vi "Adaptive Filter 2.vi"(4 "Beta":fxp<+/-,24,0>, 6 "Noise":T1, 8 "Weights":refnum<k21>="Filter Weights 0", 9 "Taps":refnum<k21>="Filter Taps 0", 11 "Input":fxp<+/-,16,2>) -> (3 "Error Out":fxp<+/-,16,2> format="%.16g")   [LabVIEW 2013]
uses:
  <vilib>/Platform/TimedLoop/XDataNode/timing_clust.ctl
  <vilib>/Platform/TimedLoop/XDataNode/nitl_modes.ctl
  <vilib>/Platform/TimedLoop/XDataNode/wakeup.ctl
  <vilib>/rvi/Emulation/niFpgaSctlEmulationGetInTimedLoop.vi
  <vilib>/rvi/Emulation/niFpgaEmulationReportErrorSimple.vi
  <vilib>/rvi/Emulation/niFpgaGetClockAttributes.vi
  <vilib>/rvi/Emulation/niFpgaCriticalErrorInLSC.vi
  <vilib>/rvi/DataTransferAndStorage/Container/Common/niFpgaContainerExecOnDevCompGetState.vi
  <vilib>/rvi/Memory/Memory_Emulation/nirvimemoryFastEmulationFpgaImpl.vi
  <instcachedir>/0/nirvimemoryFastEmulationFpgaImpl_5FBAB50466BC4C939F684F8805638BFC.lvgen/nirvimemoryFastEmulationFpgaImpl_5FBAB50466BC4C939F684F8805638BFC_002.vi
  <vilib>/rvi/DataTransferAndStorage/Container/Common/niFpgaContainerGetUniqueNameForEmu.vi
  <vilib>/rvi/Memory/Memory_Emulation/niFpgaMemoryEmulationCacheClearOnFirstRun.vi
  <vilib>/rvi/Memory/Memory_Emulation/nirvimemoryEmulationManagerCache_MakeExclusive.vi
  <vilib>/rvi/Memory/Memory_Emulation/niFpgaMemoryEmulationValidateCache.vi
  <vilib>/rvi/Memory/Memory_Emulation/nirvimemoryEmulationManagerCache_ReleaseExclusive.vi
  <vilib>/rvi/Memory/Memory_Emulation/nirvimemoryEmulationManagerCache_InsertValue.vi
  <vilib>/Utility/error.llb/Clear Errors.vi
  <vilib>/rvi/Memory/Memory_Emulation/nirvimemoryEmulationManagerCache_GetValue.vi
  <vilib>/rvi/Memory/Memory_Emulation/nirvimemoryEmulationManagerCache_SetValue.vi
  <vilib>/rvi/Emulation/niFpgaSctlEmulationResourceMgr.vi
  <vilib>/Platform/TimedLoop/XDataNode/XDataNode.xnode
  <vilib>/rvi/DataTransferAndStorage/Container/XNode/niFpgaContainer.xnode
  <vilib>/rvi/Memory/Memory_Emulation/niFpgaMemoryEmulationRefIn.vi
  <vilib>/Platform/TimedLoop/XDataNode/XDNodeRunTimeDep.lvlib
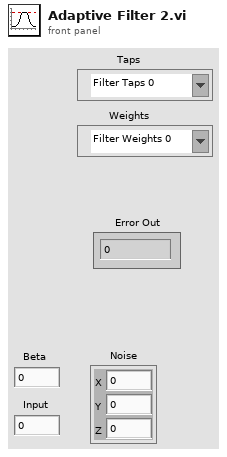
[diagram p1: front panel]
types:
  T1 = cluster{"X":fxp<+/-,16,2>, "Y":fxp<+/-,16,2>, "Z":fxp<+/-,16,2>}
  T2 = typedef "XDNodeRunTimeDep.lvlib/timing_clust.ctl" = cluster{"Expected End [f-1]":u64, "Actual End [f-1]":u64, "Finished Late? [f-1]":bool, "Expected End [i-1]":u64, "Actual End [i-1]":u64, "Finished Late? [i-1]":bool, "Expected Start [i]":u64, "Actual Start [i]":u64, "Expected Start [f]":u64, "Actual Start [f]":u64, "Source Name":string, "Structure Name":string, "Period":i64, "Deadline":i64, "Offset":i64, "Start":i64, "Priority":i32, "Timeout":i32, "Mode":T3, "Wakeup Reason":T4, "Error":errorcluster, "Source Type":string, "Secondary Source Type":string, "Global End Time":u64, "Global Start Time":u64, "Frame Duration":u64, "Iteration Duration":u64, "Assigned CPU":i32, "I/O Scan Engine Mode":u32}
  T3 = typedef "XDNodeRunTimeDep.lvlib/nitl_modes.ctl" = enum32{"No Change", "Process missed periods, maintain original phase", "Discard missed periods, maintain original phase", "Process missed periods, ignore original phase", "Discard missed periods, ignore original phase"}
  T4 = typedef "XDNodeRunTimeDep.lvlib/wakeup.ctl" = enum32{"Normal", "Aborted", "Asynchronous wakeup", "Timing source error", "Timed loop error", "Timeout"}
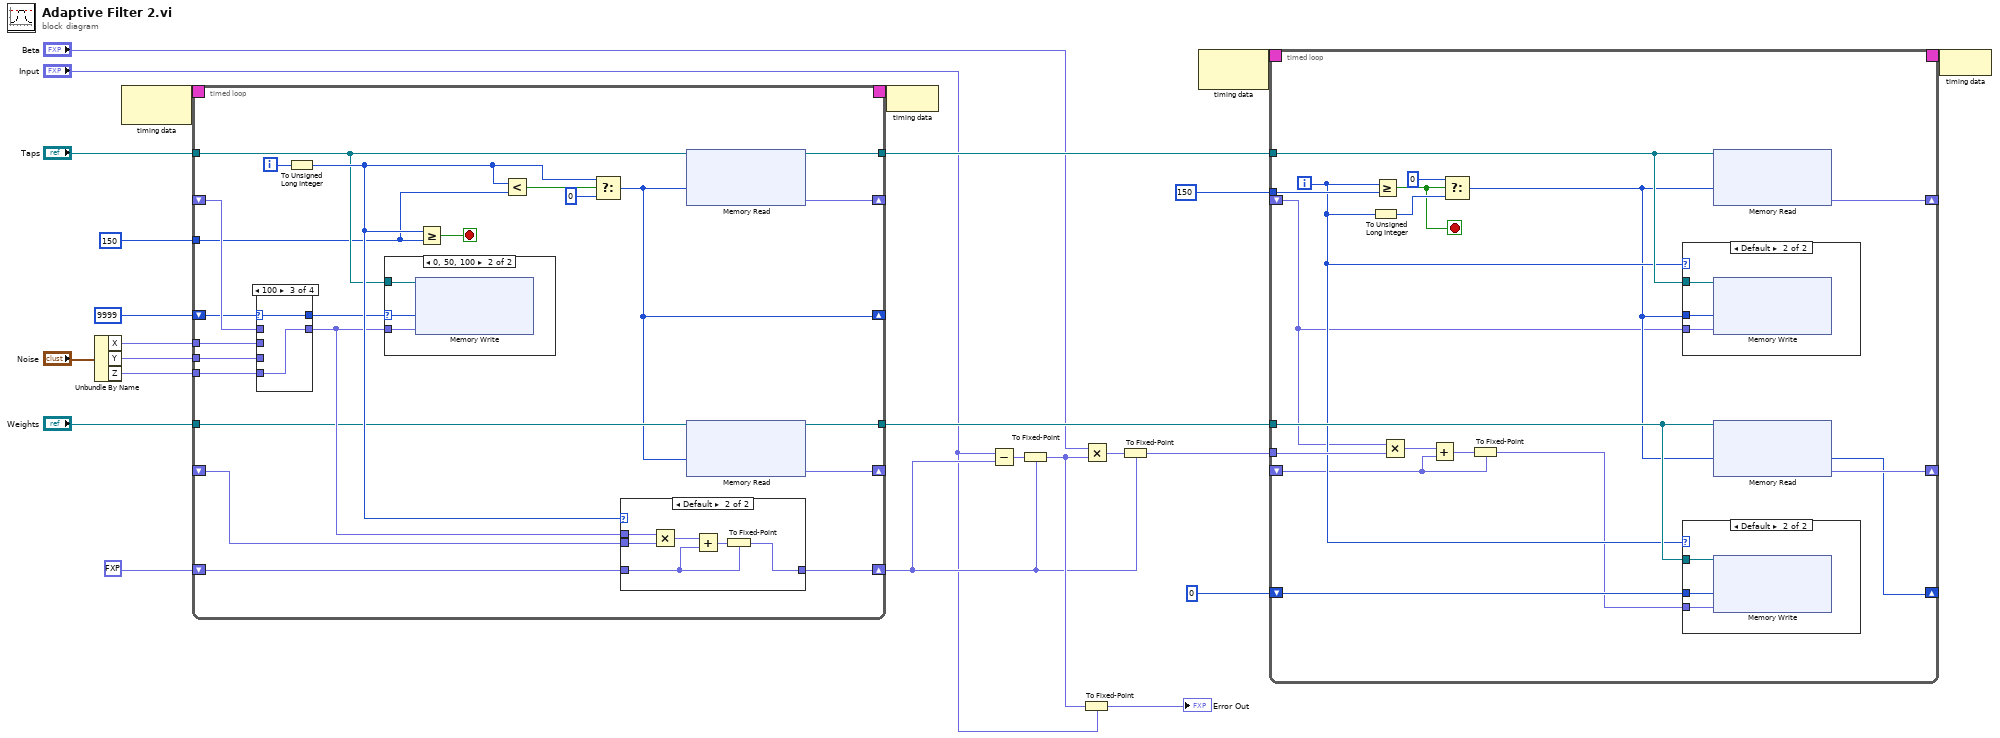
[diagram p0: block diagram]
diagram:
  n1 = Unbundle By Name("Noise") -> ("X"=w24:fxp<+/-,16,2>, "Y"=w23:fxp<+/-,16,2>, "Z"=w22:fxp<+/-,16,2>)
  n2 = node-c288() -> (w15:T2)  [unwired: 1 in]
  n3 = timed-loop {
    tunnel: "Taps" -> [w31]
    tunnel: w24 -> [w48]
    tunnel: w23 -> [w47]
    tunnel: w22 -> [w46]
    tunnel: "Weights" -> [w28]
    shift-right: [w44] -> w2
    shift-left: fxp<+/-,33,5> 0.0 ("x+y") -> [w45]
    tunnel: [w41] -> w11
    tunnel: [w42] -> w18
    timing: w15 -> [_]
    timing-out: [_] -> w14
    shift-right: [w40] -> _
    shift-left: _ -> [w36]
    shift-right: [w27] -> _
    shift-left: _ -> [w39]
    shift-right: [w26] -> _
    shift-left: u32 9999 -> [w35]
    tunnel: u32 150 ("y") -> [w29]
    i -> [w37]
    stop <- w43 stop-if-true
    n4 = case shown="100" w35 {
      selector: w35 -> [w59 w61 w63 w65]
      tunnel: w36 -> [_ _ _ w66]
      tunnel: w48 -> [w60 _ _ _]
      tunnel: w47 -> [_ w62 _ _]
      tunnel: w46 -> [_ _ w64 _]
      tunnel: [w60 w62 w64 w66] -> w30
      tunnel: [w59 w61 w63 w65] -> w32
      frame 0 {
      }
      frame 50 {
      }
      frame 100 {
      }
      frame Default {
      }
    }
    n5 = To Unsigned Long Integer(number=w37) -> (unsigned 32bit integer=w33:u32)
    n6 = case shown="0, 50, 100" w32 {
      selector: w32 -> [_ w49]
      tunnel: w31 -> [_ w51]
      tunnel: w30 -> [_ w50]
      frame Default {
      }
      frame 0, 50, 100 {
        n7 = xnode ("Memory Write")("Address"=w49, "Data"=w50, "Memory In"=w51) -> ()  [unwired: 1 out]
      }
    }
    n8 = Greater Or Equal?(x=w33, y=w29) -> (x >= y?=w43:bool)
    n9 = Less?(x=w33, y=w29) -> (x < y?=w34:bool)
    n10 = Select(t=w33, s=w34, f=u32 0) -> (s? t:f=w26:u32)
    n11 = case shown="Default" w33 {
      tunnel: w45 -> [w52 w56]
      tunnel: [w52 w55] -> w44
      tunnel: w39 -> [_ w54]
      tunnel: w30 -> [_ w53]
      frame 0 {
      }
      frame Default {
        n12 = Multiply(x=w53, y=w54) -> (x*y=w58:fxp<+/-,32,4>)
        n13 = Add(x=w58, y=w56) -> (x+y=w57:fxp<+/-,34,6>)
        n14 = To Fixed-Point(fixed-point type=w56, number=w57) -> (fixed-point=w55:fxp<+/-,33,5>)
      }
    }
    n15 = xnode ("Memory Read")("Address"=w26, "Memory In"=w31) -> ("Data"=w40:fxp<+/-,16,2>, "Memory Out"=w41:refnum<k21>)
    n16 = xnode ("Memory Read")("Address"=w26, "Memory In"=w28) -> ("Data"=w27:fxp<+/-,16,2>, "Memory Out"=w42:refnum<k21>)
  }
  n17 = node-c288(w14) -> ()
  n18 = Subtract(x="Input", y=w2) -> (x-y=w20:fxp<+/-,34,6>)
  n19 = To Fixed-Point(fixed-point type=w2, number=w20) -> (fixed-point=w19:fxp<+/-,33,5>)
  n20 = To Fixed-Point(fixed-point type="Input", number=w19) -> (fixed-point=→"Error Out":fxp<+/-,16,2>)
  n21 = Multiply(x="Beta", y=w19) -> (x*y=w17:fxp<+/-,57,5>)
  n22 = To Fixed-Point(fixed-point type=w2, number=w17) -> (fixed-point=w16:fxp<+/-,33,5>)
  n23 = node-c288() -> (w13:T2)  [unwired: 1 in]
  n24 = timed-loop {
    tunnel: w11 -> [w76]
    tunnel: w18 -> [w80]
    tunnel: w16 -> [w85]
    timing: w13 -> [_]
    timing-out: [_] -> w12
    tunnel: 150 ("y") -> [w83]
    shift-right: [w81] -> _
    shift-left: _ -> [w73]
    shift-right: [w79] -> _
    shift-left: _ -> [w70]
    shift-right: [w74] -> _
    shift-left: u32 0 ("t") -> [w78]
    i -> [w75]
    stop <- w69 stop-if-true
    n25 = To Unsigned Long Integer(number=w75) -> (unsigned 32bit integer=w77:u32)
    n26 = Greater Or Equal?(x=w75, y=w83) -> (x >= y?=w69:bool)
    n27 = Multiply(x=w73, y=w85) -> (x*y=w84:fxp<+/-,49,7>)
    n28 = Add(x=w84, y=w70) -> (x+y=w72:fxp<+/-,49,7>)
    n29 = Select(t=u32 0, s=w69, f=w77) -> (s? t:f=w74:u32)
    n30 = To Fixed-Point(fixed-point type=w70, number=w72) -> (fixed-point=w71:fxp<+/-,16,2>)
    n31 = case shown="Default" w75 {
      tunnel: w76 -> [_ w88]
      tunnel: w73 -> [_ w87]
      tunnel: w74 -> [_ w86]
      frame 0 {
      }
      frame Default {
        n32 = xnode ("Memory Write")("Address"=w86, "Data"=w87, "Memory In"=w88) -> ()  [unwired: 1 out]
      }
    }
    n33 = case shown="Default" w75 {
      tunnel: w80 -> [_ w91]
      tunnel: w71 -> [_ w90]
      tunnel: w78 -> [_ w89]
      frame 0 {
      }
      frame Default {
        n34 = xnode ("Memory Write")("Address"=w89, "Data"=w90, "Memory In"=w91) -> ()  [unwired: 1 out]
      }
    }
    n35 = xnode ("Memory Read")("Address"=w74, "Memory In"=w76) -> ("Data"=w81:fxp<+/-,16,2>)  [unwired: 1 out]
    n36 = xnode ("Memory Read")("Address"=w74, "Memory In"=w80) -> ("Data"=w79:fxp<+/-,16,2>)  [unwired: 1 out]
  }
  n37 = node-c288(w12) -> ()
